vi "Module Loop.vi"(8 "error in (no error)":errorcluster, 11 "Git Updater Module in":refnum<class "Git Updater Module.lvclass">) -> (0 "error out":errorcluster, 3 "Git Updater Module out":refnum<class "Git Updater Module.lvclass">)   [LabVIEW 2020, in "VolatusGUI.lvlib" / "Git Updater Module.lvclass"]
uses:
  Git Updater Module.lvclass
  C:/dev/lv20CE/relink/lv-volatus/Volatus/Module/Module.lvclass
  Volatus/Module/Module.lvclass/Module.ctl
  Volatus/MessageQ/MessageQ.lvclass/MessageQ.ctl
  Git Path Status Value/Git Path Status Value.lvclass
  Git Path Status Value/Git Path Status Value.lvclass/Git Path Status Value.ctl
  Volatus/Module/Module.lvclass
  Git Updater Module.lvclass/Git Updater Module.ctl
  GUI Info.ctl
  <vilib>/Utility/error.llb/Error Cluster From Error Code.vi
  lv-promises/Promises/Promise/Promise.lvclass
  Volatus/MessageQ/MessageQ.lvclass
  GUI Helper/GUI Helper.lvclass
  Volatus/VolatusAPI/VolatusAPI.lvclass
  C:/dev/lv20CE/relink/lv-volatus/VolatusGUI/Git Updater Module/Git Updater Module.lvclass
  VolatusGUI.lvlib
panel:
  in  "Revert":bool
  in  "Push":bool
  in  "Commit":bool
  in  "Refresh":bool
  in  "Pull":bool
  in  "Tags":i32(listbox)
  in  "Branches":i32(listbox)
  out "Current Tag":string
  out "Current Branch":string
  out "Commit Hash":string
  out "Remote Status":string
  out "Local Status":string
  # "Double-click a branch or tag to change to that version."
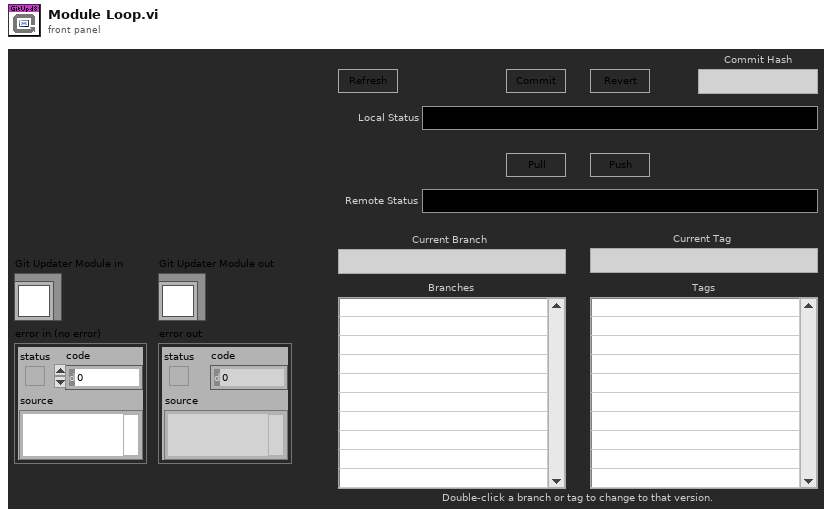
[diagram p1: front panel]
types:
  T1 = enum32{"Invalid", "Standard", "Closed", "Hidden", "Minimized", "Maximized"}
  T2 = typedef "VolatusGUI.lvlib/GUI Info.ctl" = cluster{"Color":u32, "Name":string}
  T3 = cluster{"New Branch":string, "Paths":string[], "Commit Message":string}
  T4 = enum8{"Enabled", "Disabled", "Disabled and Grayed Out"}
  T5 = typedef "VolatusGUI.lvlib/Git Updater Module.lvclass/Git Info.ctl" = cluster{"Commit":string, "Branch":string, "Tag":string, "Branches":string[], "Tags":string[], "Clean":bool, "State":T6}
  T6 = typedef "GIT-API-for-LabVIEW.lvlib/GIT-api.lvclass/GIT-Repository States.ctl" = enum16{"up-to-date", "behind", "ahead", "diverged", "unpublished", "detached", "unknown"}
  T7 = typedef "VolatusGUI.lvlib/Git Updater Module.lvclass/Path Status.ctl" = cluster{"Index":T8, "Work Tree":T8, "Path":string, "Orig Path":string}
  T8 = typedef "VolatusGUI.lvlib/Git Updater Module.lvclass/Status.ctl" = enum16{"UNKNOWN", "Unmodified", "Modified", "Added", "Deleted", "Renamed", "Unmerged", "Untracked", "Ignored"}
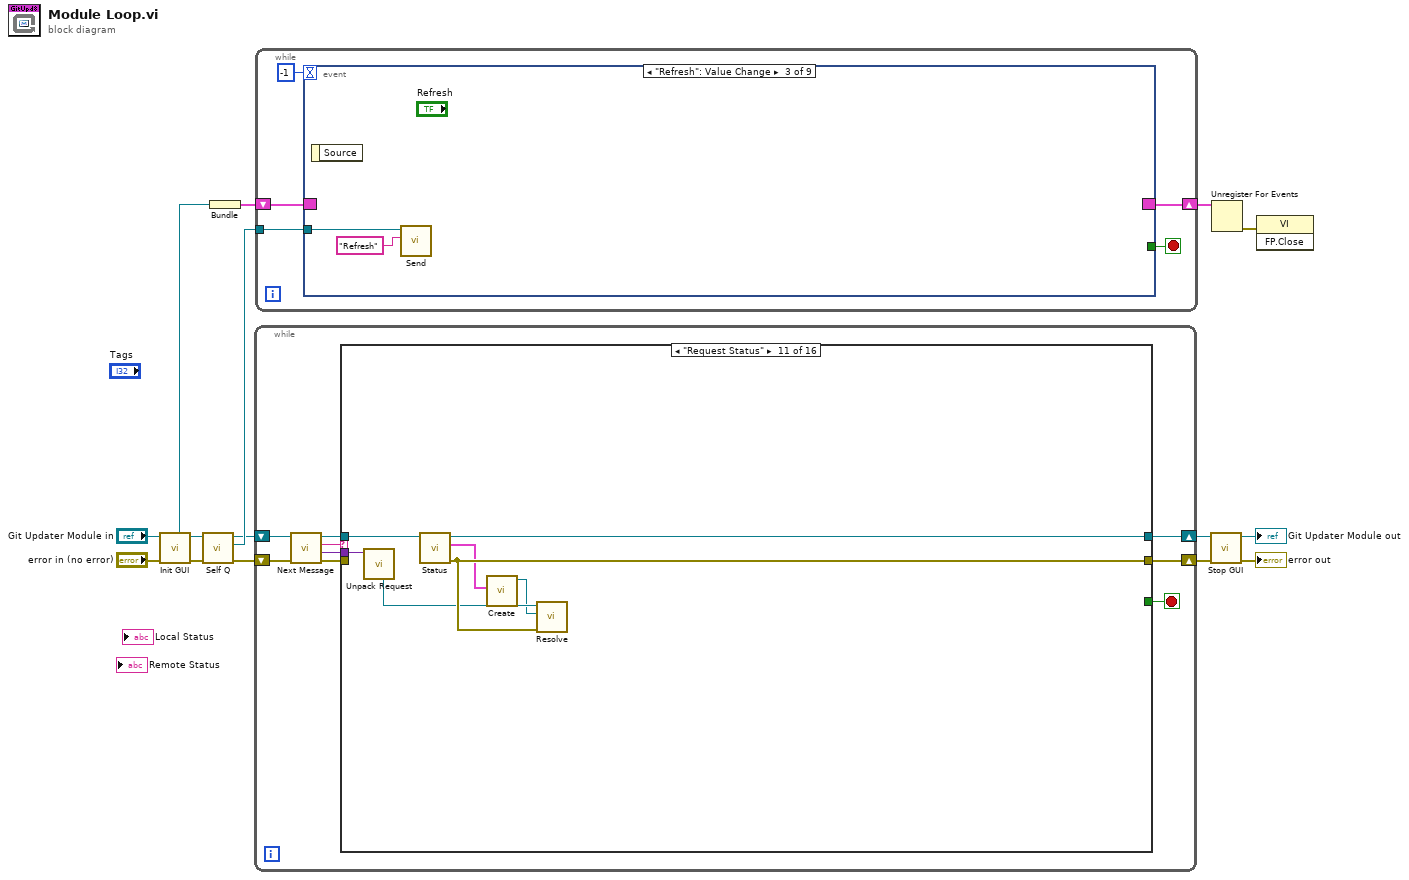
[diagram p0: block diagram]
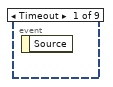
[diagram p2: hidden frame]
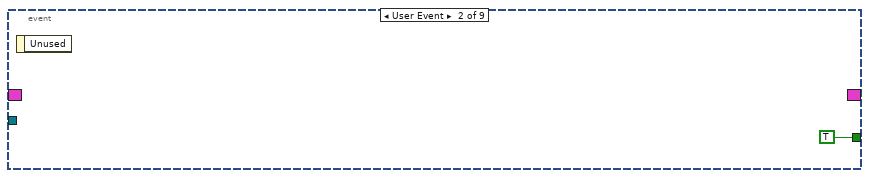
[diagram p3: hidden frame]
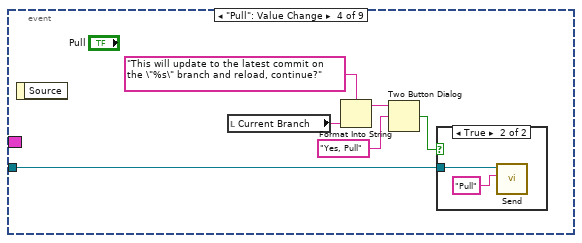
[diagram p4: hidden frame]
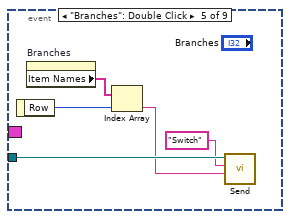
[diagram p6: hidden frame]
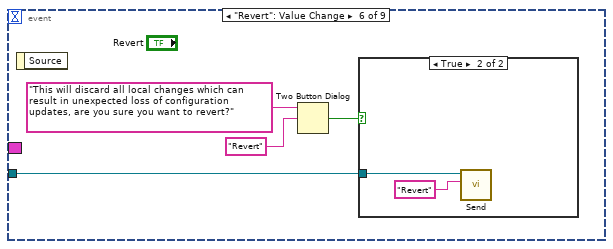
[diagram p7: hidden frame]
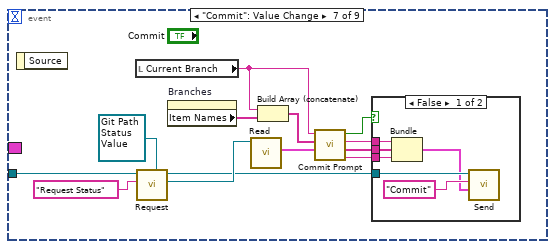
[diagram p9: hidden frame]
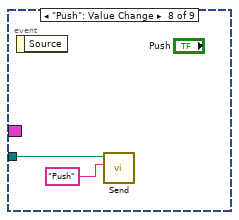
[diagram p11: hidden frame]
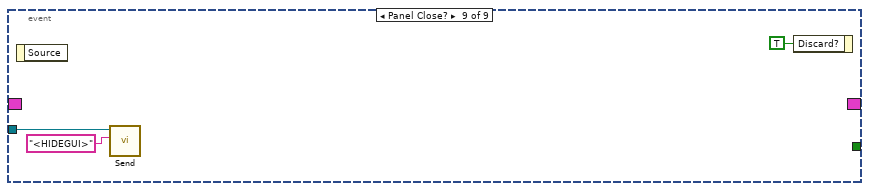
[diagram p12: hidden frame]
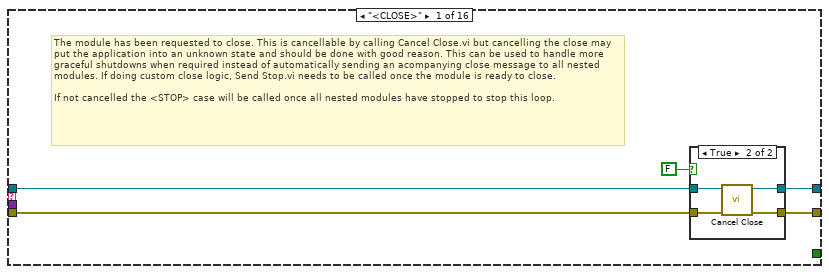
[diagram p13: hidden frame]
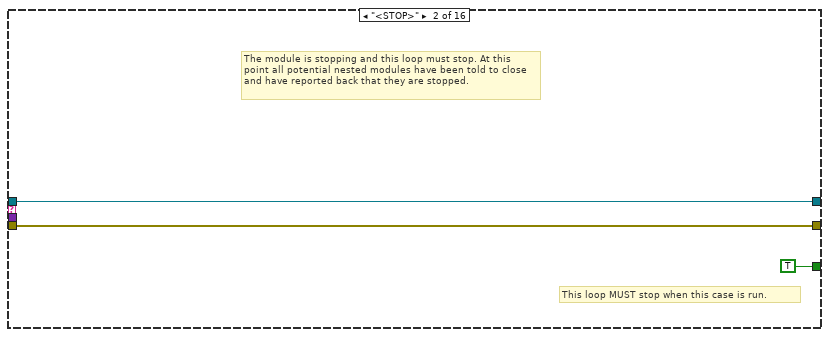
[diagram p15: hidden frame]
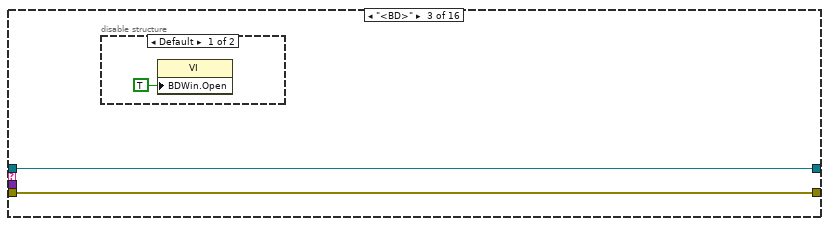
[diagram p16: hidden frame]
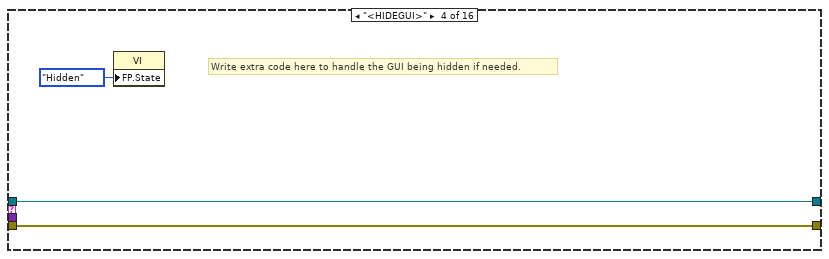
[diagram p18: hidden frame]
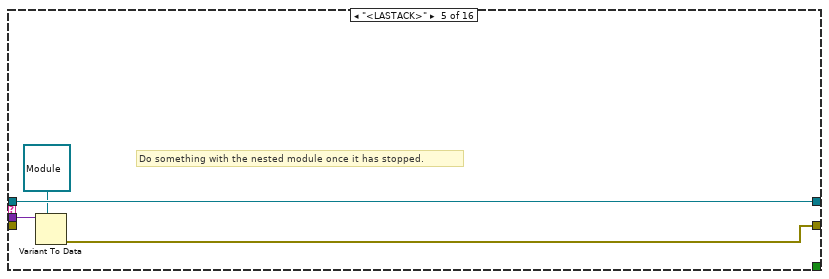
[diagram p19: hidden frame]
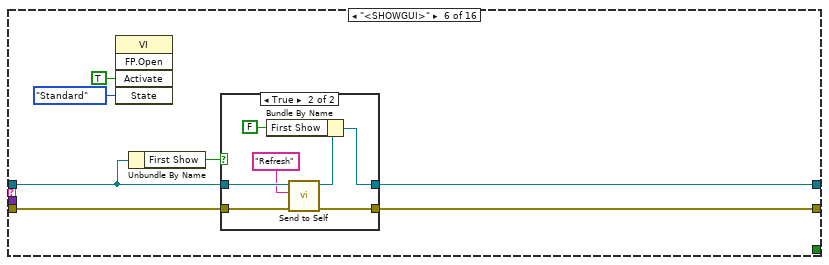
[diagram p20: hidden frame]
diagram:
  n1 = call "Init GUI.vi"("Module in"="Git Updater Module in") -> ("Module out"=w7:refnum<class "Git Updater Module.lvclass">, "Event Reg"=w12:refnum<event-registration>)  [unwired: 9 in]
  n2 = call "Self Q.vi"("Module in"=w7) -> ("Self Q"=w6:refnum<class "MessageQ.lvclass">, "Module out"=w5:refnum<class "Git Updater Module.lvclass">)  [unwired: 9 in]
  n3 = Bundle("Event Reg"=w12) -> (w8:cluster{"Event Reg":refnum<event-registration>})  [unwired: 1 in]
  n4 = while {
    shift-right: [w17] -> w10
    shift-left: w5 -> [w22]
    shift-right: [w16] -> w11
    shift-left: "error in (no error)" -> [w21]
    stop <- w15 stop-if-true
    n5 = call "Next Message.vi"("error in (no error)"=w21, "Module in"=w22) -> ("error out"=w20:errorcluster, "Data"=w14:variant, "ID"=w19:string, "Module out"=w18:refnum<class "Git Updater Module.lvclass">)  [unwired: 6 in]
    n6 = case shown="\"Request Status\"" w19 {
      tunnel: w20 -> [w25 w35 w37 w41 _ w53 w63 w74 w104 w123 _ _ w167 w180 _ w206]
      tunnel: w18 -> [w26 w36 w38 w42 w46 w48 w64 w75 w102 w122 w135 w141 w165 w178 w196 w204]
      tunnel: [w24 w36 w38 w42 w46 w49 w64 w71 w101 w119 w134 w138 w162 w175 w190 w203] -> w17
      tunnel: [w23 w35 w37 w41 w43 w50 w63 w72 w103 w118 w136 w137 w164 w177 w188 w205] -> w16
      tunnel: [_ TRUE _ _ _ _ _ _ _ _ _ _ _ _ _ _] -> w15
      tunnel: w14 -> [_ _ _ _ w45 _ _ _ _ _ w133 w143 _ _ w195 _]
      frame "<CLOSE>" {
        # "The module has been requested to close. This is cancellable by calling Cancel Close.vi but cancelling the close may put the application into an unknown state and should be done with good reason. This can be used to handle more graceful shutdowns when required instead of automatically sending an acompanying close message to all nested modules. If doing custom close logic, Send Stop.vi needs to be called once the module is ready to close.\n\nIf not cancelled the <STOP> case will be called once all nested modules have stopped to stop this loop."
        n7 = case shown="True" FALSE {
          tunnel: w25 -> [w28 w33]
          tunnel: [w28 w32] -> w23
          tunnel: w26 -> [w29 w31]
          tunnel: [w29 w30] -> w24
          frame False {
          }
          frame True {
            n8 = call "Cancel Close.vi"("error in (no error)"=w33, "Module in"=w31) -> ("error out"=w32:errorcluster, "Module out"=w30:refnum<class "Git Updater Module.lvclass">)  [unwired: 8 in]
          }
        }
      }
      frame "<STOP>" {
        # "This loop MUST stop when this case is run."
        # "The module is stopping and this loop must stop. At this point all potential nested modules have been told to close and have reported back that they are stopped."
      }
      frame "<BD>" {
        n9 = disable-structure shown="Default" {
          frame condition #0 (active) {
            n10 = property class="VI"("BDWin.Open"=TRUE ("Block Diagram Window:Open")) -> ()  [unwired: 2 in, 2 out]
          }
          frame condition #1 {
          }
        }
      }
      frame "<HIDEGUI>" {
        # "Write extra code here to handle the GUI being hidden if needed."
        n11 = property class="VI"("FP.State"=T1."Hidden" ("Front Panel Window:State")) -> ()  [unwired: 2 in, 2 out]
      }
      frame "<LASTACK>" {
        # "Do something with the nested module once it has stopped."
        n12 = Variant To Data(type=refnum<class "Module.lvclass"> refnum ("Volatus:Module"), Variant=w45) -> (error out=w43:errorcluster)  [unwired: 1 in, 1 out]
      }
      frame "<SHOWGUI>" {
        n13 = invoke class="VI" method="FP.Open"("Activate"=TRUE ("Activate?"), "State"=T1."Standard") -> ()  [unwired: 3 in, 5 out]
        n14 = Unbundle By Name(w48) -> ("First Show"=w47:bool)
        n15 = case shown="True" w47 {
          tunnel: w53 -> [w54 w62]
          tunnel: [w54 w61] -> w50
          tunnel: [w55 w57] -> w49
          tunnel: w48 -> [w55 w59]
          frame False {
          }
          frame True {
            n16 = call "Send to Self.vi"("error in (no error)"=w62, "Message ID"="Refresh", "Module in"=w59) -> ("error out"=w61:errorcluster, "Module out"=w60:refnum<class "Git Updater Module.lvclass">)  [unwired: 7 in]
            n17 = Bundle By Name(cluster=w60, "First Show"=FALSE) -> (w57:refnum<class "Git Updater Module.lvclass">)
          }
        }
      }
      frame "<TIMEOUT>" {
        # "No message for this module was received in time"
      }
      frame "Initialize" {
        n18 = Bundle By Name(cluster=w75, "First Show"=TRUE) -> (w67:refnum<class "Git Updater Module.lvclass">)
        n19 = control-ref of="This VI"() -> (w66:refnum<vi>)
        n20 = call "Launch as Nested.vi"("GUI Info (Default)"=T2 {"Color"=4547941, "Name"="Git Updater"}, "error in (no error)"=w74, "GUI"=w66, "Parent in"=w67) -> ("error out"=w69:errorcluster, "Parent"=w68:refnum<class "Git Updater Module.lvclass">)  [unwired: 5 in, 1 out]
        n21 = call "Send to Self.vi"("error in (no error)"=w69, "Message ID"="Refresh", "Module in"=w68) -> ("error out"=w72:errorcluster, "Module out"=w71:refnum<class "Git Updater Module.lvclass">)  [unwired: 7 in]
      }
      frame "Refresh" {
        n22 = flat-sequence {
          tunnel: w102 -> [w111]
          tunnel: w104 -> [w112]
          tunnel: [w112] -> w77
          tunnel: [w111] -> w76
          tunnel: [w116] -> w103
          tunnel: [w114] -> w101
          tunnel: [w113] -> w92
          tunnel: w77 -> [w117]
          tunnel: w76 -> [w115]
          frame #0 {
            w106 = -1 ("Tags")
            w107 = string[] [] ("Item Names")
            w105 = ""
            w108 = "Refreshing..." ("Local Status")
            w109 = u32 13816530
            w110 = T4."Disabled and Grayed Out" ("Disabled")
            n23 = local write "Commit Hash"(w105) -> ()
            n24 = local write "Current Branch"(w105) -> ()
            n25 = local write "Current Tag"(w105) -> ()
            n26 = property on="Branches" class="LstBox (strict)"("Item Names"=w107, "Value"=w106) -> ()  [unwired: 2 in, 2 out]
            n27 = property on="Tags" class="LstBox (strict)"("Item Names"=w107, "Value"=w106) -> ()  [unwired: 2 in, 2 out]
            n28 = property on="Revert" class="Bool"("DisabledEnum"=w110) -> ()  [unwired: 2 in, 2 out]
            n29 = property on="Local Status" class="Str"("Value"=w108, "Text.TextColor"=w109) -> ()  [unwired: 2 in, 2 out]
            n30 = property on="Remote Status" class="Str"("Value"=w108, "Text.TextColor"=w109) -> ()  [unwired: 2 in, 2 out]
            n31 = property on="Commit" class="Bool"("DisabledEnum"=w110) -> ()  [unwired: 2 in, 2 out]
            n32 = property on="Pull" class="Bool"("DisabledEnum"=w110) -> ()  [unwired: 2 in, 2 out]
            n33 = property on="Push" class="Bool"("DisabledEnum"=w110) -> ()  [unwired: 2 in, 2 out]
          }
          frame #1 {
            n34 = call "Read Info.vi"("error in (no error)"=w117, "Git Updater Module in"=w115) -> ("error out"=w116:errorcluster, "Git Info"=w113:T5, "Git Updater Module out"=w114:refnum<class "Git Updater Module.lvclass">)  [unwired: 7 in]
          }
        }
        n35 = call "Build Status.vi"("Git Info"=w92) -> ("Remote Color"=w88:u32, "Remote Status"=w85:string, "Local Color"=w86:u32, "Local Status"=w87:string, "Commit"=w84:T4, "Revert"=w81:T4, "Pull"=w83:T4, "Push"=w82:T4)  [unwired: 3 in]
        n36 = Unbundle By Name(w92) -> ("Commit"=w100:string, "Branches"=w99:string[], "Branch"=w90:string, "Tags"=w91:string[], "Tag"=w89:string)
        "Current Branch" <- w90
        "Current Tag" <- w89
        n37 = property on="Revert" class="Bool"("DisabledEnum"=w81) -> ()  [unwired: 2 in, 2 out]
        n38 = property on="Local Status" class="Str"("Value"=w87, "Text.TextColor"=w86) -> ()  [unwired: 2 in, 2 out]
        n39 = property on="Remote Status" class="Str"("Value"=w85, "Text.TextColor"=w88) -> ()  [unwired: 2 in, 2 out]
        n40 = property on="Commit" class="Bool"("DisabledEnum"=w84) -> ()  [unwired: 2 in, 2 out]
        n41 = property on="Pull" class="Bool"("DisabledEnum"=w83) -> ()  [unwired: 2 in, 2 out]
        n42 = property on="Push" class="Bool"("DisabledEnum"=w82) -> ()  [unwired: 2 in, 2 out]
        n43 = Search 1D Array(1D array=w99, element=w90) -> (index of element=w98:i32)  [unwired: 1 in]
        n44 = Search 1D Array(1D array=w91, element=w89) -> (index of element=w93:i32)  [unwired: 1 in]
        n45 = String Subset(string=w100, length (rest)=8 ("length (rest)")) -> (substring=w80:string)  [unwired: 1 in]
        n46 = Delete From Array(array=w99, index=w98) -> (array with subset deleted=w97:string[])  [unwired: 1 in, 1 out]
        n47 = Delete From Array(array=w91, index=w93) -> (array with subset deleted=w94:string[])  [unwired: 1 in, 1 out]
        n48 = To Upper Case(1:w80) -> (0:→"Commit Hash":string)
        n49 = property on="Branches" class="LstBox (strict)"("Item Names"=w97, "Value"=-1 ("Branches")) -> ()  [unwired: 2 in, 2 out]
        n50 = property on="Tags" class="LstBox (strict)"("Item Names"=w94, "Value"=-1 ("Branches")) -> ()  [unwired: 2 in, 2 out]
      }
      frame "Pull" {
        n51 = call "Pull.vi"("error in (no error)"=w123, "Git Updater Module in"=w122) -> ("error out"=w121:errorcluster, "Git Updater Module out"=w120:refnum<class "Git Updater Module.lvclass">)  [unwired: 8 in]
        n52 = case shown="No Error" w121 {
          selector: w121 -> [_ w128]
          tunnel: w120 -> [w127 w129]
          tunnel: [w126 w129] -> w119
          tunnel: [w124 w128] -> w118
          frame No Error {
            n53 = call "VolatusAPI.vi"("Module in"=w127) -> ("VolatusAPI"=w125:refnum<class "VolatusAPI.lvclass">, "Module out"=w126:refnum<class "Git Updater Module.lvclass">)  [unwired: 9 in]
            n54 = call "Reload Config.vi"("VolatusAPI in"=w125) -> ("error out"=w124:errorcluster)  [unwired: 9 in, 1 out]
          }
          frame Error {
            n55 = call <vilib>:"Simple Error Handler.vi"("error in (no error)"=w128) -> ()  [unwired: 4 in, 5 out]
          }
        }
      }
      frame "Request Status" {
        n56 = call "Unpack Request.vi"("Request Data"=w133) -> ("Promise"=w132:refnum<class "Promise.lvclass">)  [unwired: 8 in, 2 out]
        n57 = call "Status.vi"("Git Updater Module in"=w135) -> ("error out"=w136:errorcluster, "Path Statuses"=w131:T7[], "Git Updater Module out"=w134:refnum<class "Git Updater Module.lvclass">)  [unwired: 8 in]
        n58 = call "Create.vi"("Path Statuses"=w131) -> ("Git Path Status Value out"=w130:refnum<class "Git Path Status Value.lvclass">)  [unwired: 10 in]
        n59 = call "Resolve.vi"("error in (no error)"=w136, "Result (None)"=w130, "Promise in"=w132) -> ()  [unwired: 7 in, 2 out]
      }
      frame "Commit" {
        n60 = Variant To Data(type=T3 {"New Branch"="", "Paths"=[], "Commit Message"=""} ("output cluster"), Variant=w143) -> (data=w140:T3, error out=w139:errorcluster)  [unwired: 1 in]
        n61 = case shown="No Error" w139 {
          selector: w139 -> [_ w160]
          tunnel: w141 -> [w151 w161]
          tunnel: w140 -> [w152 _]
          tunnel: [w144 w161] -> w138
          tunnel: [w146 w160] -> w137
          frame No Error {
            n62 = Unbundle(w152) -> ("New Branch"=w150:string, "Paths"=w149:string[], "Commit Message"=w148:string)
            n63 = call "Commit.vi"("New Branch (None)"=w150, "Message"=w148, "Paths"=w149, "Git Updater Module in"=w151) -> ("error out"=w147:errorcluster, "Git Updater Module out"=w145:refnum<class "Git Updater Module.lvclass">)  [unwired: 6 in]
            n64 = case shown="No Error" w147 {
              selector: w147 -> [w157 w158]
              tunnel: [w156 w158] -> w146
              tunnel: w145 -> [w155 w159]
              tunnel: [w154 w159] -> w144
              frame No Error {
                n65 = call "Send to Self.vi"("error in (no error)"=w157, "Message ID"="Refresh", "Module in"=w155) -> ("error out"=w156:errorcluster, "Module out"=w154:refnum<class "Git Updater Module.lvclass">)  [unwired: 7 in]
              }
              frame Error {
              }
            }
          }
          frame Error {
          }
        }
      }
      frame "Push" {
        n66 = call "Push.vi"("error in (no error)"=w167, "Git Updater Module in"=w165) -> ("error out"=w166:errorcluster, "Git Updater Module out"=w163:refnum<class "Git Updater Module.lvclass">)  [unwired: 8 in]
        n67 = case shown="No Error" w166 {
          selector: w166 -> [w172 w173]
          tunnel: [w171 w173] -> w164
          tunnel: w163 -> [w170 w174]
          tunnel: [w169 w174] -> w162
          frame No Error {
            n68 = call "Send to Self.vi"("error in (no error)"=w172, "Message ID"="Refresh", "Module in"=w170) -> ("error out"=w171:errorcluster, "Module out"=w169:refnum<class "Git Updater Module.lvclass">)  [unwired: 7 in]
          }
          frame Error {
          }
        }
      }
      frame "Revert" {
        n69 = call "Revert.vi"("error in (no error)"=w180, "Git Updater Module in"=w178) -> ("error out"=w179:errorcluster, "Git Updater Module out"=w176:refnum<class "Git Updater Module.lvclass">)  [unwired: 8 in]
        n70 = case shown="No Error" w179 {
          selector: w179 -> [w185 w186]
          tunnel: [w184 w186] -> w177
          tunnel: w176 -> [w183 w187]
          tunnel: [w182 w187] -> w175
          frame No Error {
            n71 = call "Send to Self.vi"("error in (no error)"=w185, "Message ID"="Refresh", "Module in"=w183) -> ("error out"=w184:errorcluster, "Module out"=w182:refnum<class "Git Updater Module.lvclass">)  [unwired: 7 in]
          }
          frame Error {
          }
        }
      }
      frame "Switch" {
        n72 = Variant To Data(type="", Variant=w195) -> (data=w192:string, error out=w191:errorcluster)  [unwired: 1 in]
        n73 = call "Switch.vi"("error in (no error)"=w191, "Ref"=w192, "Git Updater Module in"=w196) -> ("error out"=w189:errorcluster, "Git Updater Module out"=w193:refnum<class "Git Updater Module.lvclass">)  [unwired: 7 in]
        n74 = case shown="No Error" w189 {
          selector: w189 -> [_ w201]
          tunnel: w193 -> [w200 w202]
          tunnel: [w199 w202] -> w190
          tunnel: [w197 w201] -> w188
          frame No Error {
            n75 = call "VolatusAPI.vi"("Module in"=w200) -> ("VolatusAPI"=w198:refnum<class "VolatusAPI.lvclass">, "Module out"=w199:refnum<class "Git Updater Module.lvclass">)  [unwired: 9 in]
            n76 = call "Reload Config.vi"("VolatusAPI in"=w198) -> ("error out"=w197:errorcluster)  [unwired: 9 in, 1 out]
          }
          frame Error {
          }
        }
      }
      frame Default {
        n77 = call "Report Unhandled Message ID.vi"("error in (no error)"=w206, "Module in"=w204) -> ("error out"=w205:errorcluster, "Module out"=w203:refnum<class "Git Updater Module.lvclass">)  [unwired: 8 in]
      }
    }
  }
  n78 = while {
    tunnel: w6 -> [w211]
    shift-right: [w209] -> w9
    shift-left: w8 -> [w210]
    stop <- w208 stop-if-true
    n79 = event shown="[2] \"Refresh\": Value Change" {
      selector: w210 -> [_ _ _ _ _ _ _ _ _]
      dyn-events: [_ _ _ _ _ _ _ _ _] -> w209
      timeout: -1 -> [_ _ _ _ _ _ _ _ _]
      tunnel: w211 -> [_ _ w214 w220 w225 w228 w246 w254 w256]
      tunnel: [_ TRUE _ _ _ _ _ _ _] -> w208
      event Timeout {
        n80 = event-data() -> ()  [unwired: 1 in, 1 out]
      }
      event User Event {
        n81 = event-data() -> ()  [unwired: 1 in, 1 out]
      }
      event "Refresh": Value Change {
        n82 = event-data() -> ()  [unwired: 1 in, 1 out]
        n83 = call "Send.vi"("ID"="Refresh", "MessageQ in"=w214) -> ()  [unwired: 8 in, 2 out]
      }
      event "Pull": Value Change {
        n84 = event-data() -> ()  [unwired: 1 in, 1 out]
        n85 = local read "Current Branch"() -> (w218:string)
        n86 = Format Into String(format string="This will update to the latest commit on the \"%s\" branch and reload, continue?" ("message"), w218) -> (resulting string=w217:string)  [unwired: 2 in, 1 out]
        n87 = Two Button Dialog(message=w217, 2:"Yes, Pull" ("T button name (\"OK\")")) -> (T button?=w215:bool)  [unwired: 1 in]
        n88 = case shown="True" w215 {
          tunnel: w220 -> [_ w222]
          frame False {
          }
          frame True {
            n89 = call "Send.vi"("ID"="Pull", "MessageQ in"=w222) -> ()  [unwired: 8 in, 2 out]
          }
        }
      }
      event "Branches": Double Click {
        n90 = event-data() -> ("Row"=w227:i32)  [unwired: 1 in]
        n91 = property on="Branches" class="LstBox (strict)"() -> ("Item Names"=w226:string[])  [unwired: 2 in, 2 out]
        n92 = Index Array(array=w226, index=w227) -> (element=w224:string)
        n93 = call "Send.vi"("Data"=w224, "ID"="Switch", "MessageQ in"=w225) -> ()  [unwired: 7 in, 2 out]
      }
      event "Revert": Value Change {
        n94 = event-data() -> ()  [unwired: 1 in, 1 out]
        n95 = Two Button Dialog(message="This will discard all local changes which can result in unexpected loss of configuration updates, are you sure you want to revert?", 2:"Revert") -> (T button?=w229:bool)  [unwired: 1 in]
        n96 = case shown="True" w229 {
          tunnel: w228 -> [_ w233]
          frame False {
          }
          frame True {
            n97 = call "Send.vi"("ID"="Revert", "MessageQ in"=w233) -> ()  [unwired: 8 in, 2 out]
          }
        }
      }
      event "Commit": Value Change {
        n98 = event-data() -> ()  [unwired: 1 in, 1 out]
        n99 = local read "Current Branch"() -> (w240:string)
        n100 = call "Request.vi"("Response Type (None)"=refnum<class "Git Path Status Value.lvclass"> refnum ("VolatusGUI:Git Path Status Value.lvclass"), "ID"="Request Status", "MessageQ in"=w246) -> ("Response"=w243:refnum<class "Git Path Status Value.lvclass">, "MessageQ out"=w238:refnum<class "MessageQ.lvclass">)  [unwired: 6 in, 1 out]
        n101 = property on="Branches" class="LstBox (strict)"() -> ("Item Names"=w241:string[])  [unwired: 2 in, 2 out]
        n102 = call "Read.vi"("Git Path Status Value in"=w243) -> ("Path Statuses"=w242:T7[])  [unwired: 10 in]
        n103 = Build Array (concatenate)(w240, w241) -> (w239:string[])
        n104 = call "Commit Prompt.vi"("Path Statuses"=w242, "Branches"=w239, "Branch"=w240) -> ("Commit Message"=w234:string, "Paths"=w235:string[], "New Branch"=w236:string, "Cancelled"=w237:bool)  [unwired: 5 in]
        n105 = case shown="False" w237 {
          tunnel: w238 -> [w252 _]
          tunnel: w236 -> [w250 _]
          tunnel: w235 -> [w249 _]
          tunnel: w234 -> [w248 _]
          frame False {
            n106 = Bundle("New Branch"=w250, "Paths"=w249, "Commit Message"=w248) -> (w247:T3)  [unwired: 1 in]
            n107 = call "Send.vi"("Data"=w247, "ID"="Commit", "MessageQ in"=w252) -> ()  [unwired: 7 in, 2 out]
          }
          frame True {
          }
        }
      }
      event "Push": Value Change {
        n108 = event-data() -> ()  [unwired: 1 in, 1 out]
        n109 = call "Send.vi"("ID"="Push", "MessageQ in"=w254) -> ()  [unwired: 8 in, 2 out]
      }
      event Panel Close? {
        n110 = event-data() -> ()  [unwired: 1 in, 1 out]
        n111 = call "Send.vi"("ID"="<HIDEGUI>", "MessageQ in"=w256) -> ()  [unwired: 8 in, 2 out]
        n112 = event-data("Discard?"=TRUE) -> ()  [unwired: 1 in, 1 out]
      }
    }
  }
  n113 = call "Stop GUI.vi"("error in (no error)"=w11, "Module in"=w10) -> ("error out"=→"error out":errorcluster, "Module out"=→"Git Updater Module out":refnum<class "Git Updater Module.lvclass">)  [unwired: 8 in]
  n114 = Unregister For Events(event registration refnum=w9) -> (error out=w13:errorcluster)  [unwired: 1 in]
  n115 = invoke class="VI" method="FP.Close"(error in=w13) -> ()  [unwired: 2 in, 3 out]
